vi "writeToFile.vi"(8 "error in (no error)":errorcluster, 10 "New Record String":string, 11 "Handler.File in":refnum<class "Handler.File.lvclass">) -> (0 "error out":errorcluster, 3 "Handler.File out":refnum<class "Handler.File.lvclass">)   [LabVIEW 2017, in "Error Log.lvlib" / "Handler.File.lvclass"]
uses:
  Handler.File.lvclass
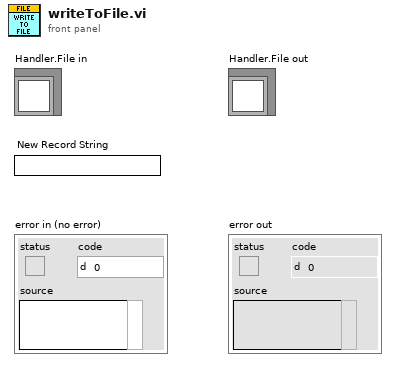
[diagram p1: front panel]
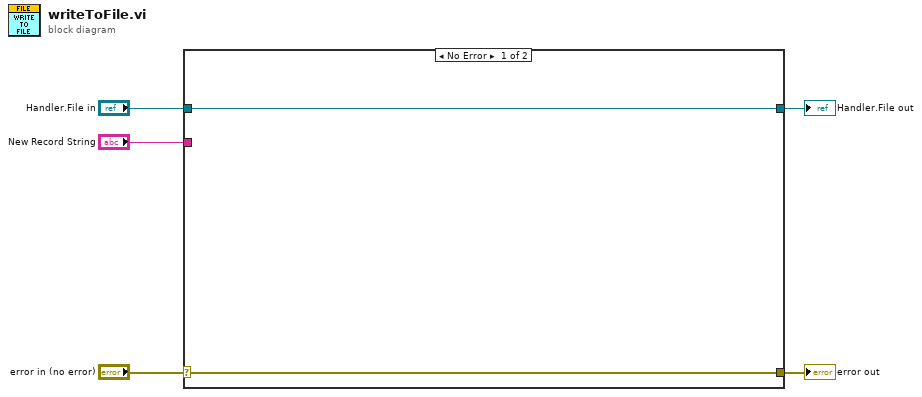
[diagram p0: block diagram]
diagram:
  n1 = case shown="No Error" "error in (no error)" {
    selector: "error in (no error)" -> [w6 w9]
    tunnel: [w6 w9] -> w4
    tunnel: [w7 w8] -> w2
    tunnel: "Handler.File in" -> [w7 w8]
    tunnel: "New Record String" -> [_ _]
    frame No Error {
    }
    frame Error {
    }
  }
  "error out" <- w4
  "Handler.File out" <- w2
